vi "Write log file.vi"(8 "error in (no error)":errorcluster) -> (0 "error out":errorcluster)   [LabVIEW 2016]
uses:
  <vilib>/Platform/TimedLoop/XDataNode/timing_clust.ctl
  <vilib>/Platform/TimedLoop/XDataNode/nitl_modes.ctl
  <vilib>/Platform/TimedLoop/XDataNode/wakeup.ctl
  <vilib>/platform/TimedLoop/XDataNode/XDataNode.xnode
  <vilib>/Platform/TimedLoop/XDataNode/XDNodeRunTimeDep.lvlib
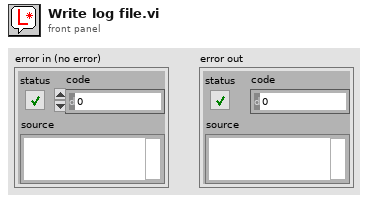
[diagram p1: front panel]
types:
  T1 = typedef "XDNodeRunTimeDep.lvlib/timing_clust.ctl" = cluster{"Expected End [f-1]":u64, "Actual End [f-1]":u64, "Finished Late? [f-1]":bool, "Expected End [i-1]":u64, "Actual End [i-1]":u64, "Finished Late? [i-1]":bool, "Expected Start [i]":u64, "Actual Start [i]":u64, "Expected Start [f]":u64, "Actual Start [f]":u64, "Source Name":string, "Structure Name":string, "Period":i64, "Deadline":i64, "Offset":i64, "Start":i64, "Priority":i32, "Timeout":i32, "Mode":T2, "Wakeup Reason":T3, "Error":errorcluster, "Source Type":string, "Secondary Source Type":string, "Global End Time":u64, "Global Start Time":u64, "Frame Duration":u64, "Iteration Duration":u64, "Assigned CPU":i32, "I/O Scan Engine Mode":u32}
  T2 = typedef "XDNodeRunTimeDep.lvlib/nitl_modes.ctl" = enum32{"No Change", "Process missed periods, maintain original phase", "Discard missed periods, maintain original phase", "Process missed periods, ignore original phase", "Discard missed periods, ignore original phase"}
  T3 = typedef "XDNodeRunTimeDep.lvlib/wakeup.ctl" = enum32{"Normal", "Aborted", "Asynchronous wakeup", "Timing source error", "Timed loop error", "Timeout"}
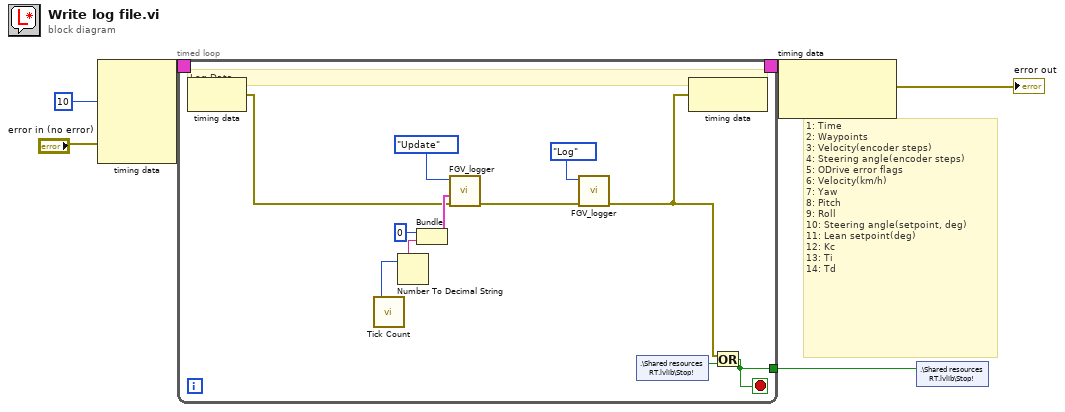
[diagram p0: block diagram]
diagram:
  # "1: Time\n2: Waypoints\n3: Velocity(encoder steps)\n4: Steering angle(encoder steps)\n5: ODrive error flags\n6: Velocity(km/h)\n7: Yaw\n8: Pitch\n9: Roll\n10: Steering angle(setpoint, deg)\n11: Lean setpoint(deg)\n12: Kc\n13: Ti\n14: Td"
  n1 = node-c288(i64 10 ("Period"), "error in (no error)") -> (w5:T1)  [unwired: 3 in]
  n2 = timed-loop {
    tunnel: [w16] -> w6
    timing: w5 -> [_]
    timing-out: [_] -> w4
    stop <- w16 stop-if-true
    # "Log Data"
    n3 = node-c288() -> (w8:errorcluster)  [unwired: 1 in]
    n4 = call "Tick Count"() -> ("Tick Count(mSec)"=w11:u32)
    n5 = Number To Decimal String(number=w11) -> (decimal integer string=w12:string)  [unwired: 1 in]
    n6 = Bundle(0, w12) -> (w14:cluster{i32, string})  [unwired: 1 in]
    n7 = call "FGV_logger.vi"("error in"=w8, 9:w14, "Command"=enum16{"Update", "Log", "Init"}."Update") -> ("error out"=w9:errorcluster)  [unwired: 8 in]
    n8 = call "FGV_logger.vi"("error in"=w9, "Command"=enum16{"Update", "Log", "Init"}."Log") -> ("error out"=w7:errorcluster)  [unwired: 9 in]
    n9 = shared-variable ".\\Shared resources RT.lvlib\\Stop!"() -> (w17:bool)  [unwired: 1 in, 1 out]
    n10 = node-c288(w7) -> ()  [unwired: 1 out]
    n11 = Or(x=w7, y=w17) -> (x .or. y?=w16:bool)
  }
  n12 = node-c288(w4) -> (→"error out":errorcluster)  [unwired: 1 out]
  n13 = shared-variable ".\\Shared resources RT.lvlib\\Stop!"(w6) -> ()  [unwired: 1 in, 1 out]
